vi "Get DDS Cur Boxing Amplitude Mv.vi"(11 "boxing":u32) -> (3 "function return":i32)   [LabVIEW 2021, in "vmmso.lvlib"]
doc: "DLL_API int WINAPI GetDDSCurBoxingAmplitudeMv(unsigned int boxing);"
uses:
  vmmso.lvlib
  vmmso.dll
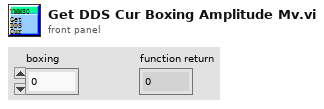
[diagram p1: front panel]
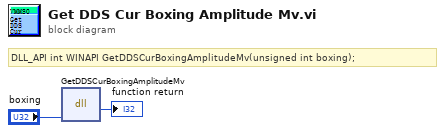
[diagram p0: block diagram]
diagram:
  # "DLL_API int WINAPI GetDDSCurBoxingAmplitudeMv(unsigned int boxing);"
  n1 = dll-call lib="D:/labviewdemo/LabviewDemo 21/vmmso/vmmso.*" fn="GetDDSCurBoxingAmplitudeMv"("boxing"="boxing") -> (→"function return":i32)  [unwired: 4 in, 2 out]
